vi "Autobalance Window.vi"() -> ()   [LabVIEW 2013]
uses:
  lib/Launcher/Launcher Actions.ctl
  lib/Launcher/NoPanelAppTypes.ctl
  lib/Data Access Objects/Metadata/Persistant DAO Actions.ctl
  lib/Global Data/Transactions/Dataset Source.ctl
  lib/Data Access Objects/Metadata/DAO Actions.ctl
  lib/Apps/App Parameters Actions.ctl
  lib/Data Access Objects/Metadata/LBCB Number.ctl
  lib/Autobalance/Autobalance Stage.ctl
  lib/Apps/Yes No Button.ctl
  lib/Autobalance/Autobalance Display Data Point.ctl
  lib/Data Access Objects/Autobalance/Autobalance Control Parameters.ctl
  lib/Data Access Objects/Metadata/Actuator Point.ctl
  lib/Apps/Colored Labels.ctl
panel:
  in  "Status Tab Control":enum32{"Data", "Advanced", "Parameters"}(tab)
  in  "Start":bool
  in  "Stop":bool
  in  "Finish":bool
  in  "L2 Control":bool caption="Control LBCB 2"
  out "Forces L1":dbl[](array[numeric]) caption="Forces & Moments"
  out "AB Diff L1":dbl[](array[numeric]) caption="Differences"
  out "Actuator DOF Labels":T1={"X1"="X1", "X2"="X2", "Y1"="Y1", "Z1"="Z1", "Z2"="Z2", "Z3"="Z3"}
  out "Forces L2":dbl[](array[numeric]) caption="Forces & Moments"
  out "AB Diff L2":dbl[](array[numeric]) caption="Differences"
  in  "L2 Label":string="LBCB 2"
  in  "L1 Label":string="LBCB 1"
  in  "L1 Control":bool caption="Control LBCB 1"
  out "Actuator DOF Labels 2":T1={"X1"="X1", "X2"="X2", "Y1"="Y1", "Z1"="Z1", "Z2"="Z2", "Z3"="Z3"}
  in  "Advanced Tabs":enum32{"LBCB 1", "LBCB 2"}(tab)
  out "Autobalance Statuses L1":T2[](array[typedef])
  out "Autobalance Statuses L2":T2[](array[typedef])
  in  "LBCB 2 Error Tolerance":T5
  in  "LBCB 1 Error Tolerance":T5
  in  "Auto Balance Control":T6={"Number of Samples"=0, "Delay After Cmd"=0, "Maximum Command"=0.0, "1/4 Linear Range"=0.5}
  # "Cmd"
  # "Servo Error"
  # "Cmd"
  # "Servo Error"
  # "(Volts)"
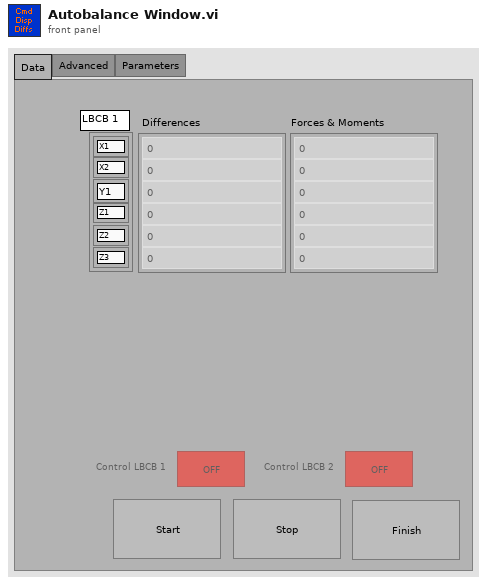
[diagram p1: front panel]
types:
  T1 = typedef "Colored Labels.ctl" = cluster{"X1":string, "X2":string, "Y1":string, "Z1":string, "Z2":string, "Z3":string}
  T2 = typedef "Autobalance Display Data Point.ctl" = cluster{"LoCmd":dbl, "LoServo":dbl, "HiCmd":dbl, "HiServo":dbl, "Autobalance Stage":T3, "IsBalanced":T4}
  T3 = typedef "Autobalance Stage.ctl" = enum16{"Coarse", "Fine", "Backing Up", "Done"}
  T4 = typedef "Yes No Button.ctl" = bool
  T5 = typedef "Actuator Point.ctl" = cluster{"X1":dbl, "X2":dbl, "Y1":dbl, "Z1":dbl, "Z2":dbl, "Z3":dbl}
  T6 = typedef "Autobalance Control Parameters.ctl" = cluster{"Number of Samples":i32, "Delay After Cmd":i32, "Maximum Command":dbl, "1/4 Linear Range":dbl}
  T7 = typedef "App Parameters Actions.ctl" = enum16{"Init", "Get", "Set"}
  T8 = typedef "Persistant DAO Actions.ctl" = enum16{"Init", "Get", "Set", "Load", "Save"}
  T9 = typedef "Number Of LBCBs.ctl" = enum16{"1", "2"}
  T10 = enum8{"Enabled", "Disabled", "Disabled and Grayed Out"}
  T11 = typedef "App Parameters.ctl" = cluster{"Monitor Loop":T12, "Ramp Time":T12, "Log Loop":T12, "TCP to DAQ":T12, "Logging Directory":path, "Log File Size (MBytes)":i64, "Volt Logging Loop":T12, "2 LBCB Archiving Mode":bool, "Fake":bool}
  T12 = typedef "Timing Parameters.ctl" = cluster{"Interval":dbl, "Rate ":dbl}
  T13 = typedef "DAO Actions.ctl" = enum16{"Init", "Get", "Set"}
  T14 = typedef "Dataset Source.ctl" = enum16{"Continuous", "Hold", "ED", "Volts", "Offsets", "Increments"}
  T15 = typedef "LBCB Number.ctl" = enum16{"LBCB1", "LBCB2"}
  T16 = typedef "Autobalance Status Data.ctl" = cluster{"IsBalanced":T4, "Autobalance Stage":T3, "High":T17, "Low":T17, "Balanced \nCmd":dbl}
  T17 = typedef "Autobalance Data Point.ctl" = cluster{"cCmd":dbl, "cServo":dbl, "pCmd":dbl, "pServo":dbl}
  T18 = typedef "NoPanelAppTypes.ctl" = enum16{"NTCP Socket", "Data Archiving", "DAQ Link", "Control Loops", "Cmd Disp Diffs", "LBCB Data", "Limits", "Mixed Mode Widget", "Offsets", "Debug"}
  T19 = typedef "Launcher Actions.ctl" = enum16{"Launch", "Stop All", "Stop", "Kill", "Running?", "Init"}
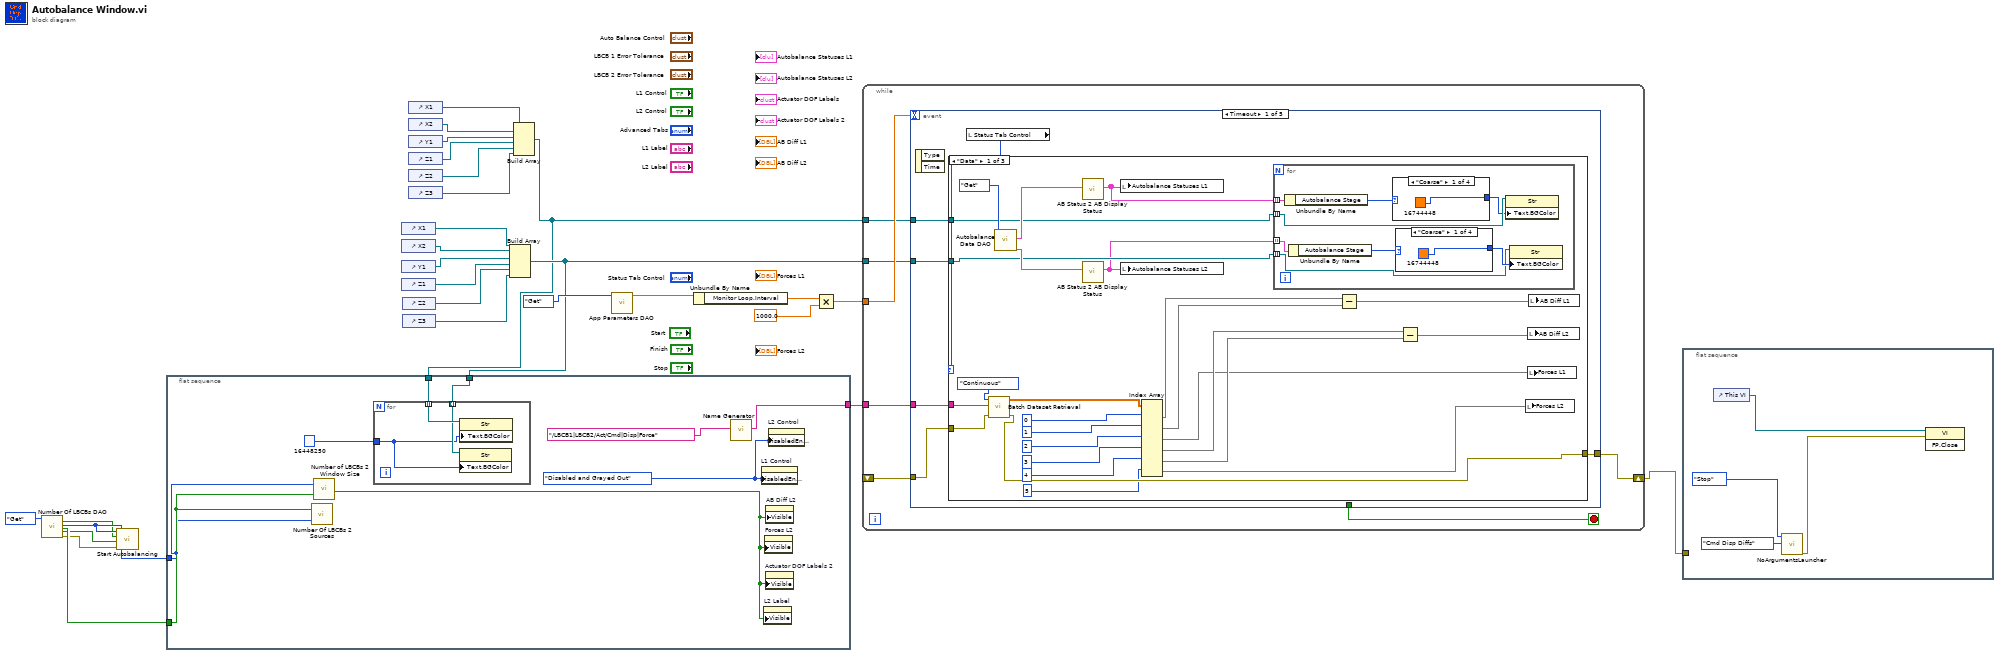
[diagram p0: block diagram]
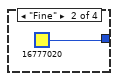
[diagram p2: hidden frame]
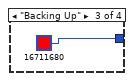
[diagram p3: hidden frame]
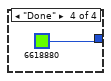
[diagram p4: hidden frame]
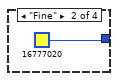
[diagram p5: hidden frame]
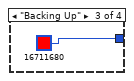
[diagram p6: hidden frame]
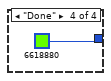
[diagram p7: hidden frame]
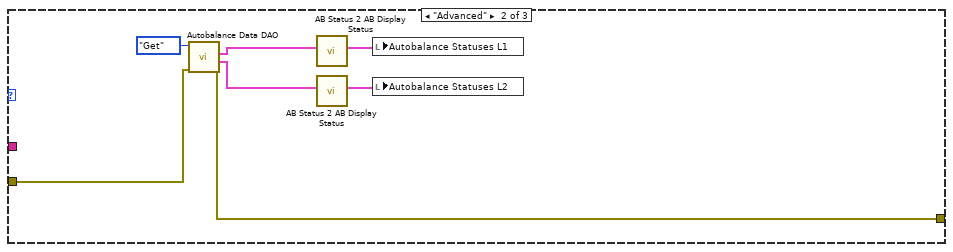
[diagram p8: hidden frame]
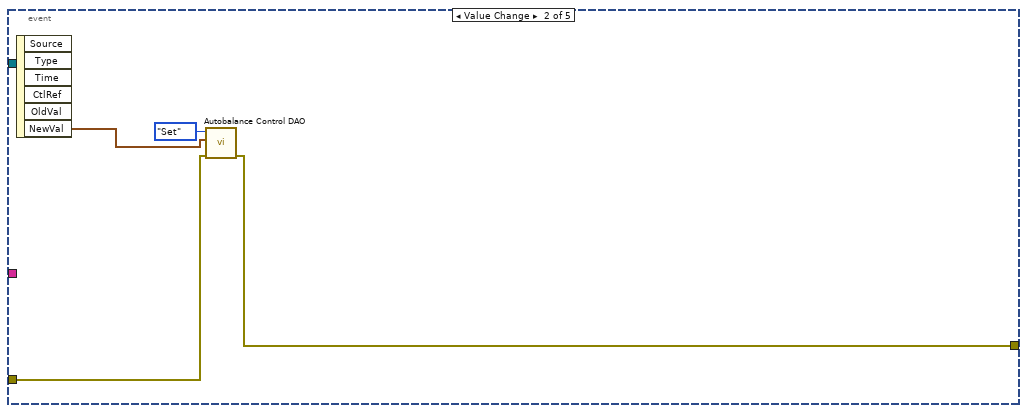
[diagram p10: hidden frame]
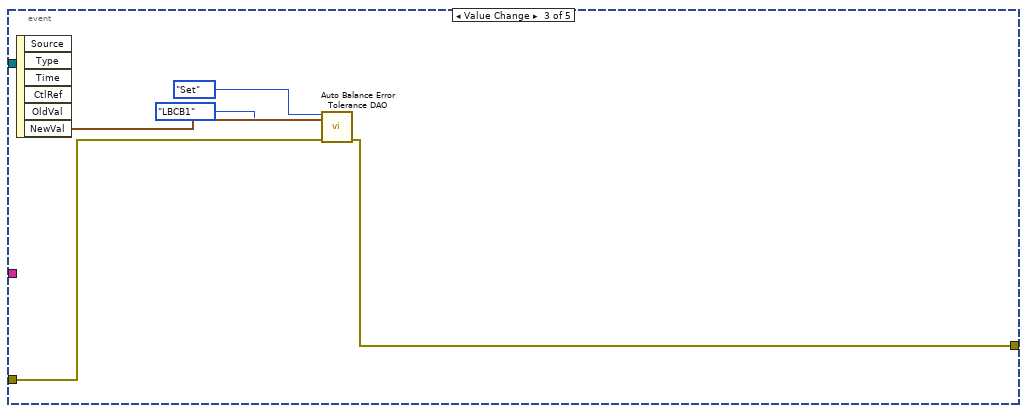
[diagram p11: hidden frame]
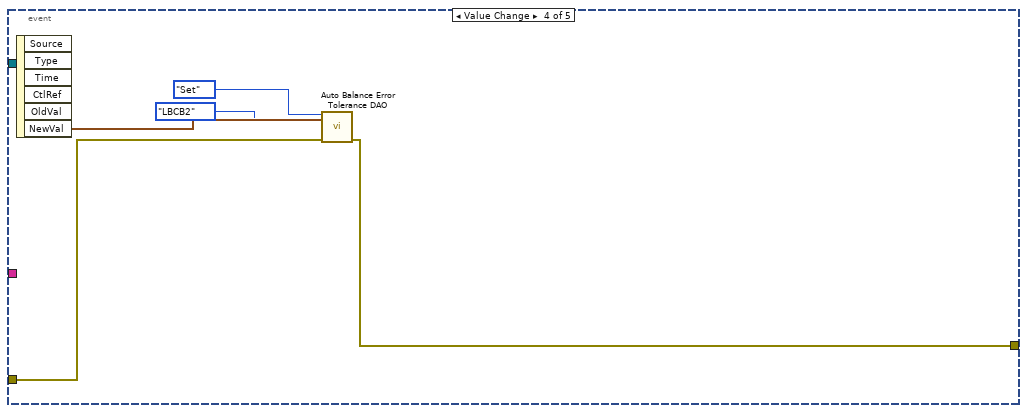
[diagram p12: hidden frame]
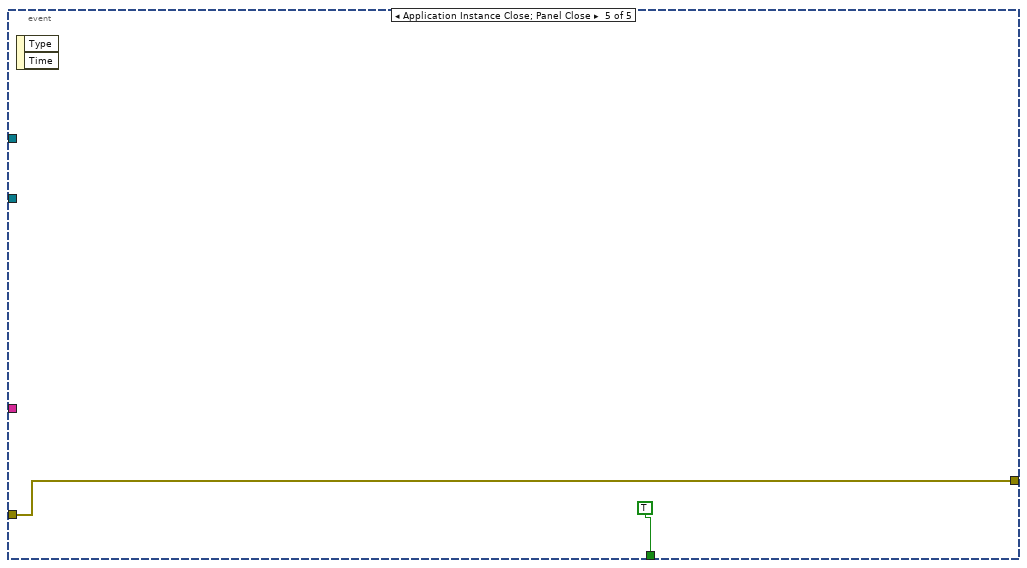
[diagram p13: hidden frame]
diagram:
  n1 = call "Number Of LBCBs DAO.vi"("Actions"=Persistant_DAO_Actions."Get") -> ("LBCB 1 Balanced Out"=w21:bool, "Number of\nLBCBs Out"=w23:T9, "Rigid Connection Out"=w25:bool, "LBCB 2 Balanced Out"=w22:bool, "error out"=w24:errorcluster)  [unwired: 13 in, 1 out]
  n2 = call "Start Autobalancing.vi"("error in (no error)"=w24, "L2 Control"=w22, "L1 Control"=w21, "Number of\nLBCBs In"=w23) -> ()  [unwired: 5 in, 3 out]
  n3 = flat-sequence {
    tunnel: w25 -> [w35]
    tunnel: w23 -> [w34]
    tunnel: [w32] -> w20
    tunnel: w2 -> [w28]
    tunnel: w1 -> [w30]
    frame #0 {
      w31 = T10."Disabled and Grayed Out" ("Disabled")
      n4 = call "Number Of LBCBs 2 Sources.vi"("Number of LBCBs"=w34, "Combined LBCBs"=w35) -> ()  [unwired: 2 out]
      n5 = call "Number of LBCBs 2 Window Size.vi"("Number of\nLBCBs Out"=w34, "Rigid Connection In"=w35) -> ("LBCB 2 Visible"=w36:bool)  [unwired: 1 in, 2 out]
      n6 = for {
        tunnel: w30 -> [w39] mode=indexing
        tunnel: u32 16448250 -> [w37]
        tunnel: w28 -> [w38] mode=indexing
        n7 = property class="Str"(reference=w38, "Text.BGColor"=w37) -> ()  [unwired: 1 in, 2 out]
        n8 = property class="Str"(reference=w39, "Text.BGColor"=w37) -> ()  [unwired: 1 in, 2 out]
      }
      n9 = call "Name Generator.vi"("Group Specifier"="/LBCB1|LBCB2/Act/Cmd|Disp|Force") -> ("Group Names"=w32:string[])  [unwired: 10 in]
      n10 = property on="L1 Control" class="Bool (strict)"("DisabledEnum"=w31) -> ()  [unwired: 2 in, 2 out]
      n11 = property on="L2 Label" class="Str"("Visible"=w36) -> ()  [unwired: 2 in, 2 out]
      n12 = property on="Forces L2" class="Arr (strict)"("Visible"=w36) -> ()  [unwired: 2 in, 2 out]
      n13 = property on="Actuator DOF Labels 2" class="Clust (strict)"("Visible"=w36) -> ()  [unwired: 2 in, 2 out]
      n14 = property on="AB Diff L2" class="Arr (strict)"("Visible"=w36) -> ()  [unwired: 2 in, 2 out]
      n15 = property on="L2 Control" class="Bool (strict)"("DisabledEnum"=w31) -> ()  [unwired: 2 in, 2 out]
    }
  }
  n16 = control-ref of="X1"() -> (w8:refnum<vi>)
  n17 = control-ref of="X2"() -> (w7:refnum<vi>)
  n18 = control-ref of="Y1"() -> (w6:refnum<vi>)
  n19 = control-ref of="Z1"() -> (w5:refnum<vi>)
  n20 = control-ref of="Z2"() -> (w4:refnum<vi>)
  n21 = control-ref of="Z3"() -> (w3:refnum<vi>)
  n22 = control-ref of="X1"() -> (w14:refnum<vi>)
  n23 = control-ref of="X2"() -> (w13:refnum<vi>)
  n24 = control-ref of="Y1"() -> (w12:refnum<vi>)
  n25 = control-ref of="Z1"() -> (w11:refnum<vi>)
  n26 = control-ref of="Z2"() -> (w10:refnum<vi>)
  n27 = control-ref of="Z3"() -> (w9:refnum<vi>)
  n28 = Build Array(w8, w7, w6, w5, w4, w3) -> (w2:refnum<vi>[])
  n29 = Build Array(w14, w13, w12, w11, w10, w9) -> (w1:refnum<vi>[])
  n30 = call "App Parameters DAO.vi"("Actions"=App_Parameters_Actions."Get" ("App Parameter Actions")) -> ("Application Timing and Logging Out"=w16:T11)  [unwired: 3 in, 7 out]
  n31 = Unbundle By Name(w16) -> ("Monitor Loop.Interval"=w19:dbl)
  n32 = Multiply(x=w19, y=1000.0) -> (x*y=w15:dbl)
  n33 = while {
    shift-right: [w44] -> w27
    shift-left: _ -> [w45]
    tunnel: w20 -> [w43]
    tunnel: w15 -> [w42]
    tunnel: w1 -> [w41]
    tunnel: w2 -> [w40]
    stop <- w46 stop-if-true
    n34 = event shown="[0] Timeout" {
      selector: _ -> [_ _ _ _ _]
      dyn-events: _ -> [_ _ _ _ _]
      timeout: w42 -> [_ _ _ _ _]
      tunnel: [_ _ _ _ TRUE] -> w46
      tunnel: w45 -> [w51 w104 w108 w113 w117]
      tunnel: [w50 w103 w107 w112 w117] -> w44
      tunnel: w43 -> [w52 _ _ _ _]
      tunnel: w41 -> [w48 _ _ _ _]
      tunnel: w40 -> [w47 _ _ _ _]
      event Timeout {
        n35 = event-data() -> ()  [unwired: 3 out]
        n36 = local read "Status Tab Control"() -> (w49:enum32{"Data", "Advanced", "Parameters"})
        n37 = case shown="\"Data\"" w49 {
          tunnel: w52 -> [w75 _ _]
          tunnel: w51 -> [w74 w98 w102]
          tunnel: [w73 w97 w102] -> w50
          tunnel: w48 -> [w55 _ _]
          tunnel: w47 -> [w54 _ _]
          frame "Data" {
            n38 = call "Batch Dataset Retrieval.vi"("Dataset Source"=Dataset_Source."Continuous", "Transactions"=w75, "error in"=w74) -> ("Data"=w72:dbl[][], "error out"=w73:errorcluster)  [unwired: 6 in]
            n39 = call "Autobalance Data DAO.vi"("DAO Actions"=DAO_Actions."Get") -> ("L2 Autobalance Out"=w57:T16[], "L1 Autobalance Out"=w58:T16[])  [unwired: 3 in, 6 out]
            n40 = call "AB Status 2 AB Display Status.vi"("Autobalance Status In"=w58) -> ("Autobalance Statuses Out"=w56:T2[])  [unwired: 10 in]
            n41 = call "AB Status 2 AB Display Status.vi"("Autobalance Status In"=w57) -> ("Autobalance Statuses Out"=w53:T2[])  [unwired: 10 in]
            n42 = local write "Autobalance Statuses L1"(w56) -> ()
            n43 = local write "Autobalance Statuses L2"(w53) -> ()
            n44 = Index Array(array=w72, index (row) #1=0 ("index"), index (row) #2=1 ("index"), index (row) #3=2 ("index"), index (row) #4=3 ("index"), index (row) #5=4 ("index"), index (row) #6=5 ("index")) -> (element #1=w67:dbl[], element #2=w66:dbl[], element #3=w63:dbl[], element #4=w65:dbl[], element #5=w64:dbl[], element #6=w62:dbl[])  [unwired: 6 in]
            n45 = for {
              tunnel: w56 -> [w86] mode=indexing
              tunnel: w55 -> [w84] mode=indexing
              tunnel: w54 -> [w79] mode=indexing
              tunnel: w53 -> [w80] mode=indexing
              n46 = Unbundle By Name(w86) -> ("Autobalance Stage"=w85:T3)
              n47 = Unbundle By Name(w80) -> ("Autobalance Stage"=w81:T3)
              n48 = case shown="\"Coarse\"" w85 {
                tunnel: [u32 16744448 u32 16777020 u32 16711680 u32 6618880] -> w83
                frame "Coarse" {
                }
                frame "Fine" {
                }
                frame "Backing Up" {
                }
                frame "Done" {
                }
              }
              n49 = case shown="\"Coarse\"" w81 {
                tunnel: [u32 16744448 u32 16777020 u32 16711680 u32 6618880] -> w82
                frame "Coarse" {
                }
                frame "Fine" {
                }
                frame "Backing Up" {
                }
                frame "Done" {
                }
              }
              n50 = property class="Str"(reference=w84, "Text.BGColor"=w83) -> ()  [unwired: 1 in, 2 out]
              n51 = property class="Str"(reference=w79, "Text.BGColor"=w82) -> ()  [unwired: 1 in, 2 out]
            }
            n52 = Subtract(x=w67, y=w66) -> (x-y=w60:dbl[])
            n53 = Subtract(x=w65, y=w64) -> (x-y=w61:dbl[])
            n54 = local write "Forces L2"(w62) -> ()
            n55 = local write "Forces L1"(w63) -> ()
            n56 = local write "AB Diff L2"(w61) -> ()
            n57 = local write "AB Diff L1"(w60) -> ()
          }
          frame "Advanced" {
            n58 = call "Autobalance Data DAO.vi"("error in (no error)"=w98, "DAO Actions"=DAO_Actions."Get") -> ("error out"=w97:errorcluster, "L2 Autobalance Out"=w99:T16[], "L1 Autobalance Out"=w100:T16[])  [unwired: 2 in, 5 out]
            n59 = call "AB Status 2 AB Display Status.vi"("Autobalance Status In"=w100) -> ("Autobalance Statuses Out"=w96:T2[])  [unwired: 10 in]
            n60 = call "AB Status 2 AB Display Status.vi"("Autobalance Status In"=w99) -> ("Autobalance Statuses Out"=w95:T2[])  [unwired: 10 in]
            n61 = local write "Autobalance Statuses L1"(w96) -> ()
            n62 = local write "Autobalance Statuses L2"(w95) -> ()
          }
          frame "Parameters" {
          }
        }
      }
      event Value Change {
        n63 = event-data() -> ("NewVal"=w105:T6)  [unwired: 6 out]
        n64 = call "Autobalance Control DAO.vi"("error in (no error)"=w104, "Autobalance Control In"=w105, "Persistent DAO Actions"=Persistant_DAO_Actions."Set") -> ("error out"=w103:errorcluster)  [unwired: 6 in, 2 out]
      }
      event Value Change {
        n65 = event-data() -> ("NewVal"=w110:T5)  [unwired: 6 out]
        n66 = call "Auto Balance Error Tolerance DAO.vi"("Auto Balance Increment Actions"=Persistant_DAO_Actions."Set", 2:w110, "LBCB Number"=LBCB_Number."LBCB1", "error in (no error)"=w108) -> ("error out"=w107:errorcluster)  [unwired: 9 in, 2 out]
      }
      event Value Change {
        n67 = event-data() -> ("NewVal"=w115:T5)  [unwired: 6 out]
        n68 = call "Auto Balance Error Tolerance DAO.vi"("Auto Balance Increment Actions"=Persistant_DAO_Actions."Set", 2:w115, "LBCB Number"=LBCB_Number."LBCB2", "error in (no error)"=w113) -> ("error out"=w112:errorcluster)  [unwired: 9 in, 2 out]
      }
      event Application Instance Close; Panel Close {
        n69 = event-data() -> ()  [unwired: 3 out]
      }
    }
  }
  n70 = flat-sequence {
    tunnel: w27 -> [_]
    frame #0 {
      n71 = control-ref of="This VI"() -> (w120:refnum<vi>)
      n72 = call "NoArgumentsLauncher.vi"("Application"=NoPanelAppTypes."Cmd Disp Diffs", "Application Launcher Actions"=Launcher_Actions."Stop") -> ("error out"=w119:errorcluster)  [unwired: 1 in, 8 out]
      n73 = invoke class="VI" method="FP.Close"(reference=w120, error in=w119) -> ()  [unwired: 1 in, 3 out]
    }
  }
